vi "Main.vi"() -> ()   [LabVIEW 2021, in "Game of Life.lvlib"]
doc: "This template is for the Queued Message Handler design pattern.\n\nThe Event Handling Loop generates messages based on user interface actions.\n\nThe Message Handling Loop processes messages generated by the Event Handling Loop, or by other messages. The messages are string values, so new messages can be added easily to the Message Cases case structure in the Message Handling Loop. Each message cluster can also provide an optional value for Message Data, which is a variant that can be converted to whatever message-specific data is required."
uses:
  Game of Life.lvlib
  <vilib>/Plug-In SDKs/InstrumentStudio SDK/InstrumentStudioPluginSDK.lvlibp/Plugin Events Enum.ctl
  controls/Data.ctl
  controls/Configuration.ctl
  controls/Game of Life.ctl
  a2cd5499-92a9-455c-b0f9-1db12e3f6067.vi
  aef85ed4-6d5b-4a62-8cd4-232f16e6ae51.vi
  a2cd5499-92a9-455c-b0f9-1db12e3f6067.vi/6651a77e-856e-4bcd-af5a-c0c13b264cc1.vi
  aef85ed4-6d5b-4a62-8cd4-232f16e6ae51.vi/331b549c-fcf8-43d9-8a1e-5b3c0091a99c.vi
  <vilib>/JDP Science/JSONtext/JSON text to Variant.vi
  <vilib>/Utility/error.llb/Error Cluster From Error Code.vi
  <vilib>/JDP Science/JSONtext/Variant to JSON Text.vi
  <vilib>/JDP Science/JSONtext/LVClass Serializer/JSONtext LVClass Serializer.lvclass
  <vilib>/ErrorRing/Error Ring.xnode
  <vilib>/Plug-In SDKs/InstrumentStudio SDK/InstrumentStudioPluginSDK.lvlibp/Plugin Session.lvclass
  <vilib>/Plug-In SDKs/InstrumentStudio SDK/InstrumentStudioPluginSDK.lvlibp
panel:
  in  "Tab Control":enum32{"Game Panel", "Events"}(tab)
  in  "IS Project":bool
  in  "Start":bool
  out "game of life":T1(graph)
  out "generation":u32 caption="Generation"
  in  "update interval":u32=250 caption="Update interval (msec)" min=50
  in  "height":u32=100 caption="Board height" min=10
  in  "width":u32=100 caption="Board width" min=10
  out "Project Path":path
  out "Event Record":i32(listbox)
  in  "Session Id":u64
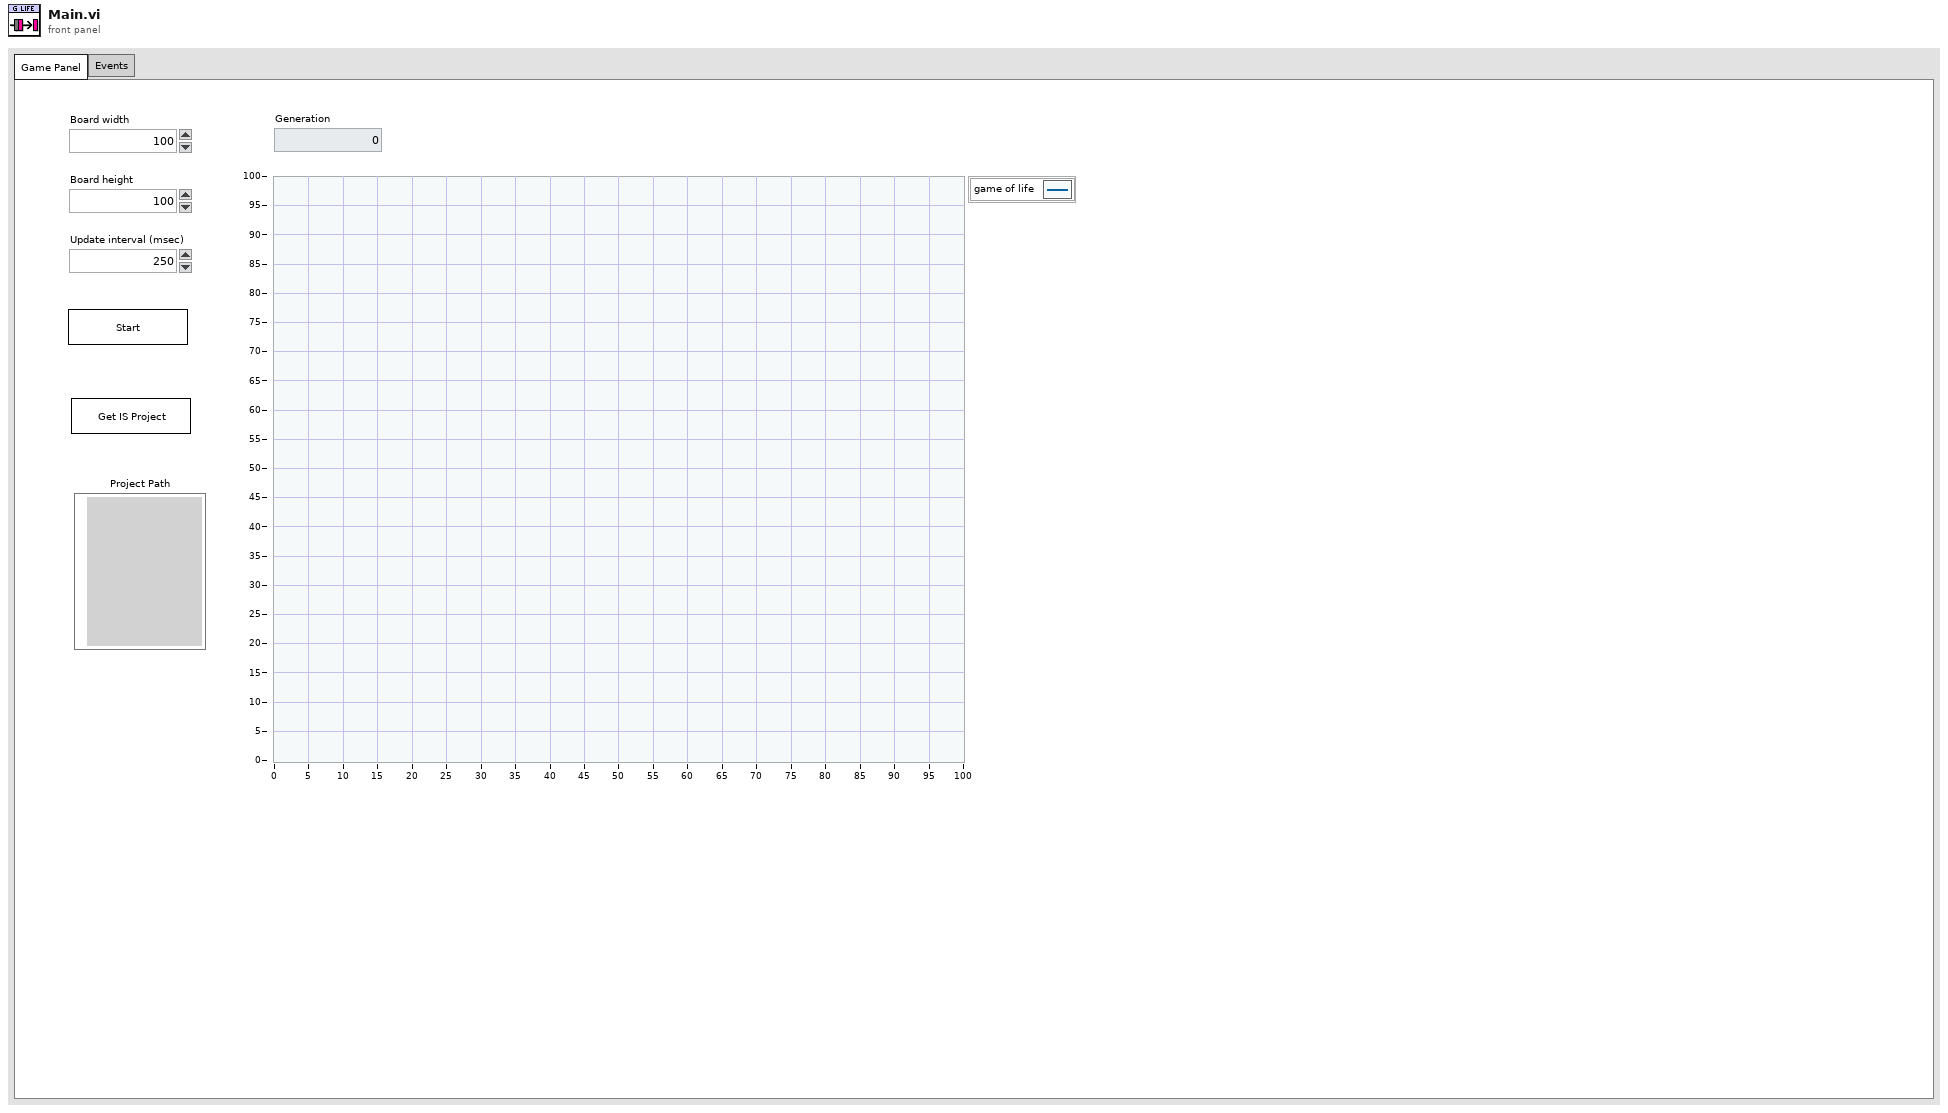
[diagram p1: front panel]
types:
  T1 = typedef "Game of Life.lvlib/Game of Life.ctl" = cluster{"x_data":dbl[], "y_data":dbl[]}
  T2 = typedef "Game of Life.lvlib/Data.ctl" = cluster{"Height":u32, "Width":u32, "Update Interval":u32, "Generation":u32, "Run?":bool, "Cells":bool[][], "Project Path":path}
  T3 = typedef "InstrumentStudioPluginSDK.lvlibp/Plugin Events Enum.ctl" = enum16{"Shutdown", "Project Saved", "Stop All Outputs"}
  T4 = typedef "InstrumentStudioPluginSDK.lvlibp/Event Registration Refnum.ctl" = refnum<event-registration>
  T5 = typedef "Game of Life.lvlib/All Message Queues.ctl" = cluster{"UI":refnum<queue>}
  T6 = cluster{"Event Refnum":T4, "Event Registration Refnum":refnum<event-registration>}
  T7 = typedef "Game of Life.lvlib/Configuration.ctl" = cluster{"Height":u32, "Width":u32, "Update Interval":u32, "Project Path":path}
  T8 = enum8{"Enabled", "Disabled", "Disabled and Grayed Out"}
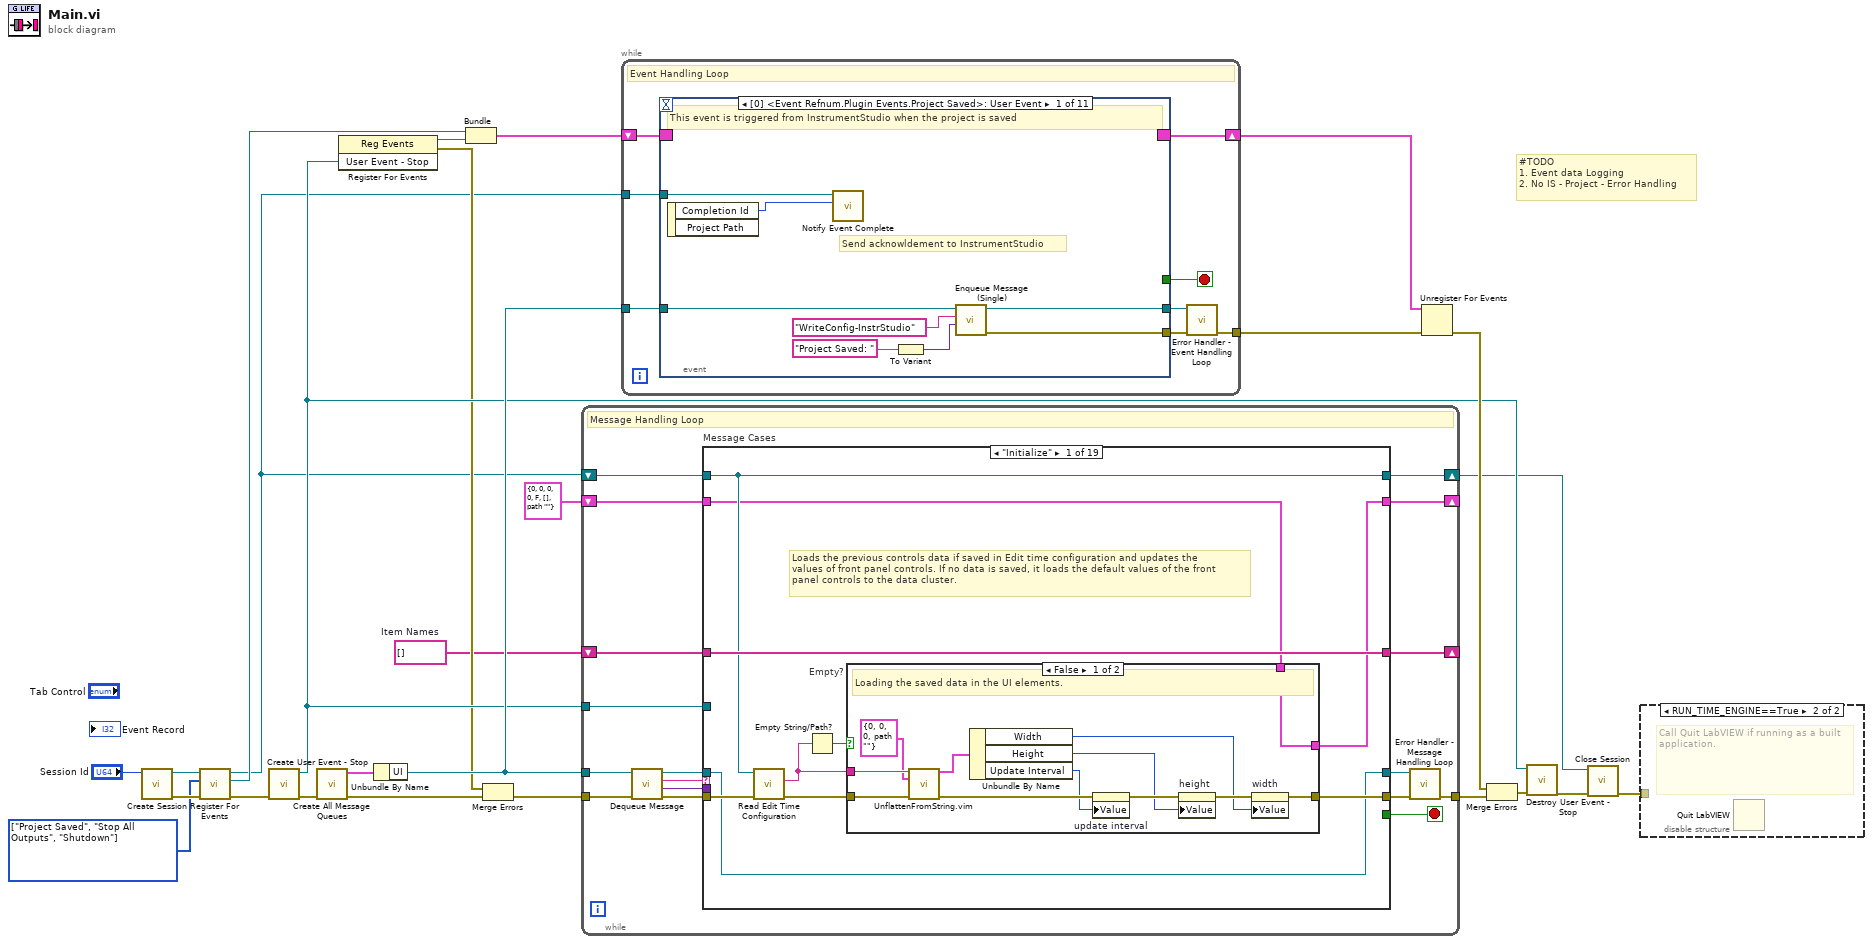
[diagram p0: block diagram]
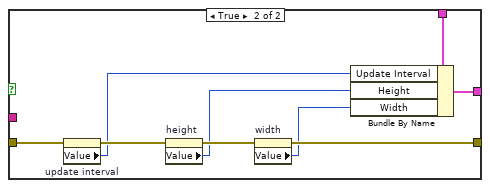
[diagram p3: hidden frame]
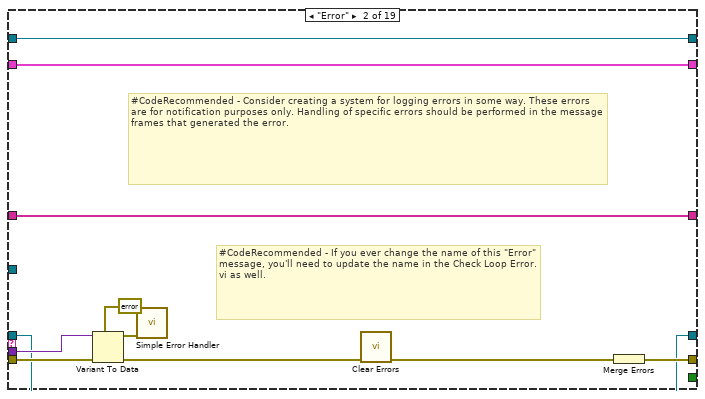
[diagram p4: hidden frame]
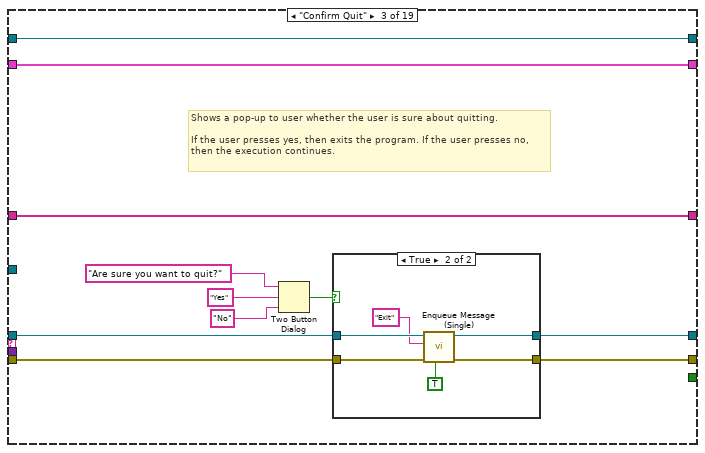
[diagram p5: hidden frame]
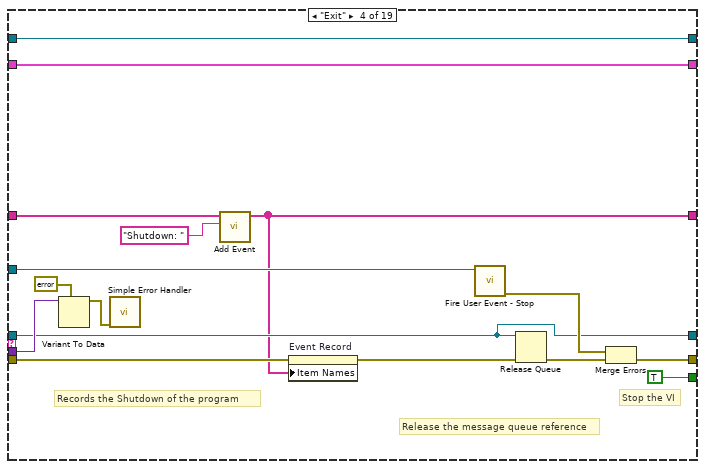
[diagram p7: hidden frame]
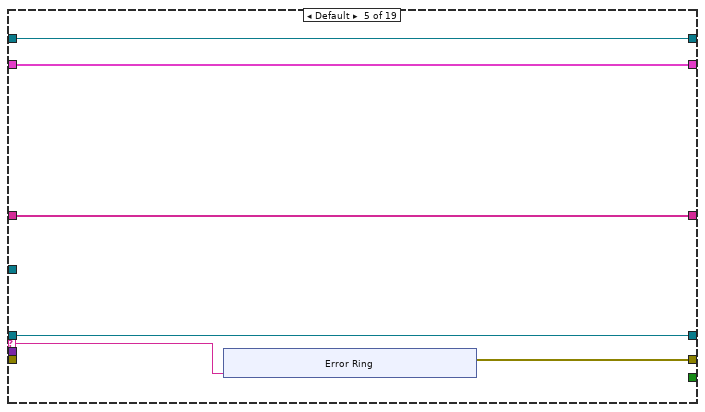
[diagram p8: hidden frame]
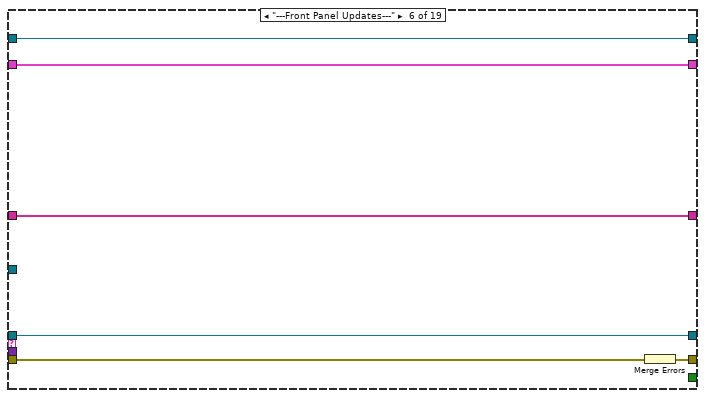
[diagram p9: hidden frame]
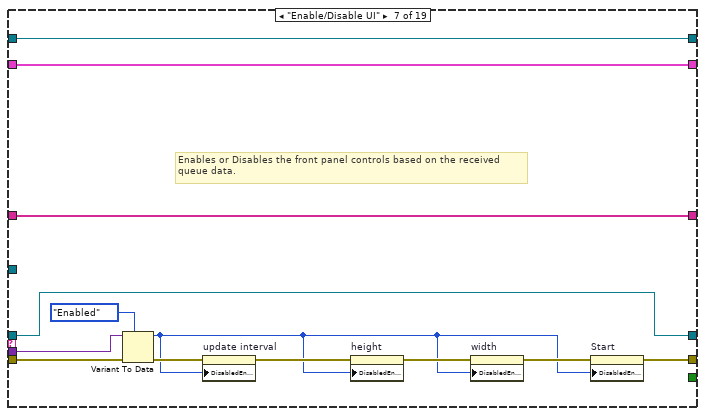
[diagram p10: hidden frame]
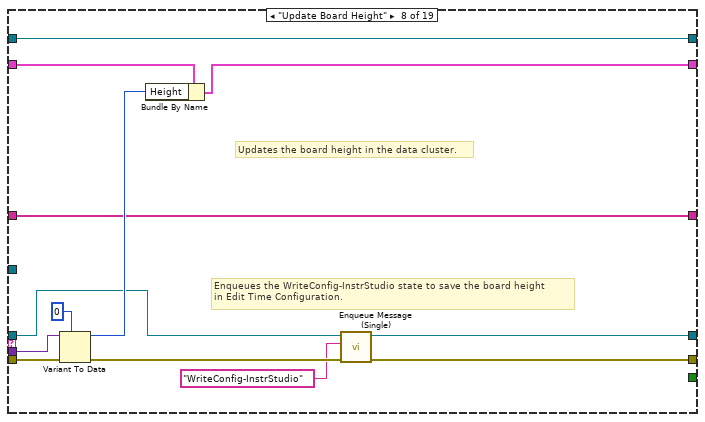
[diagram p11: hidden frame]
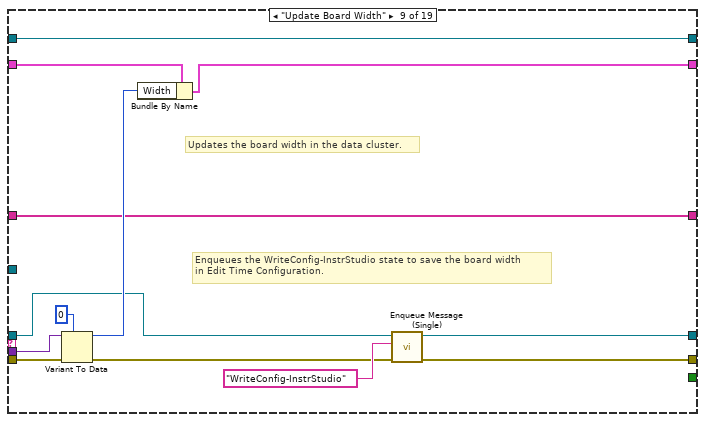
[diagram p12: hidden frame]
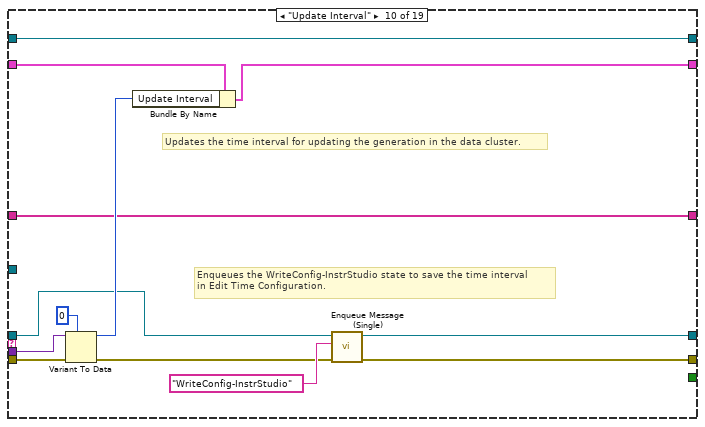
[diagram p13: hidden frame]
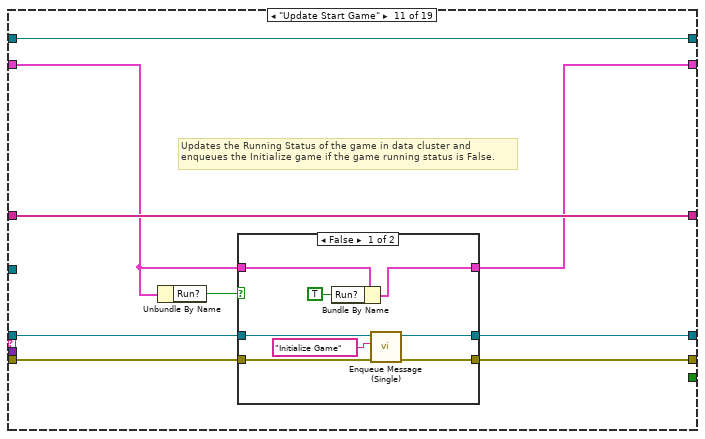
[diagram p14: hidden frame]
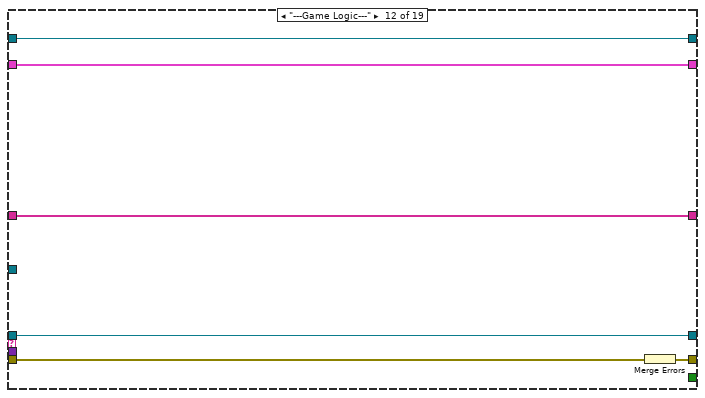
[diagram p16: hidden frame]
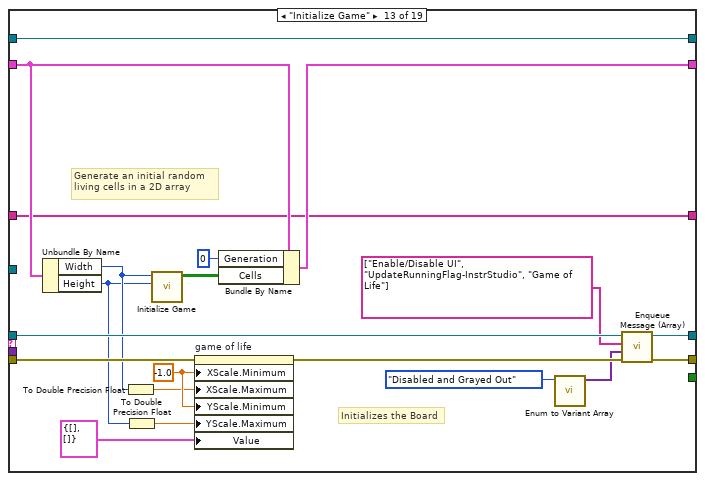
[diagram p17: hidden frame]
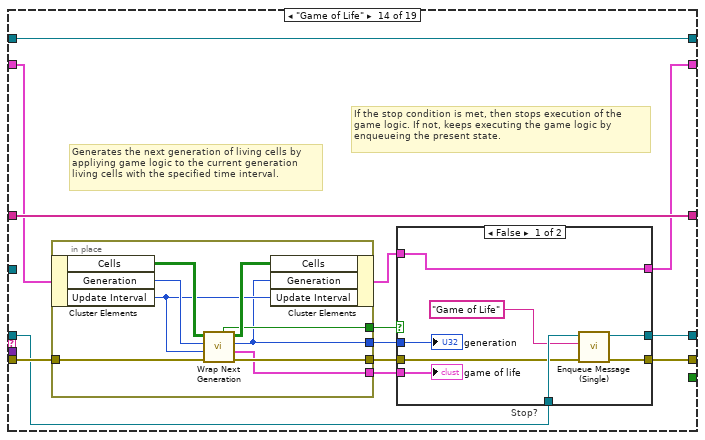
[diagram p18: hidden frame]
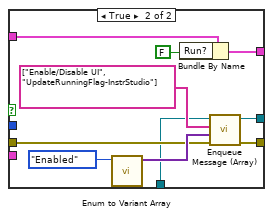
[diagram p19: hidden frame]
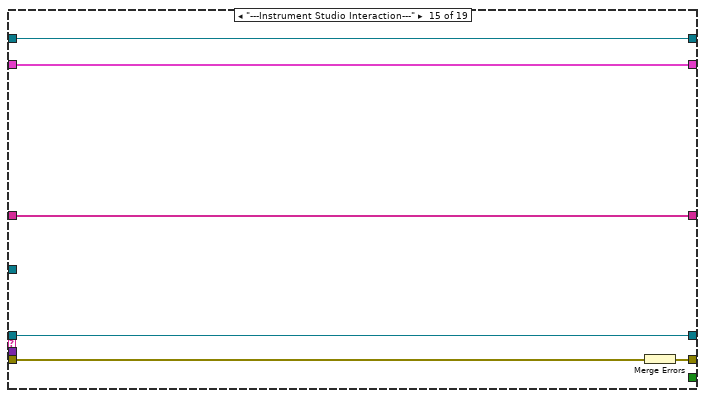
[diagram p20: hidden frame]
diagram:
  w1 = string[] []  # Item Names
  w10 = T3[] [enum."Project Saved", enum."Stop All Outputs", enum."Shutdown"] items=["Shutdown", "Project Saved", "Stop All Outputs"] ("Events To Register")
  # "#TODO\n1. Event data Logging\n2. No IS - Project - Error Handling"
  n1 = call <vilib>:"Create Session.vi"("Session Id"="Session Id") -> ("error out"=w13:errorcluster, "Session out"=w11:refnum<class "Plugin Session.lvclass">)  [unwired: 6 in, 3 out]
  n2 = call <vilib>:"Register For Events.vi"("error in (no error)"=w13, "Events To Register"=w10, "Session in"=w11) -> ("error out"=w12:errorcluster, "Event Refnum"=w7:T4, "Session out"=w3:refnum<class "Plugin Session.lvclass">)  [unwired: 6 in]
  n3 = call "Create User Event - Stop.vi"("error in (no error)"=w12) -> ("error out"=w22:errorcluster, "User Event - Stop"=w17:refnum<user-event>)  [unwired: 9 in]
  n4 = call "Create All Message Queues.vi"("error in (no error)"=w22) -> ("error out"=w26:errorcluster, "Message Queues out"=w25:T5)  [unwired: 9 in]
  n5 = register-events(w17) -> (reference out=w9:refnum<event-registration>, error out=w15:errorcluster)  [unwired: 2 in]
  n6 = Unbundle By Name(w25) -> ("UI"=w23:refnum<queue>)
  n7 = Bundle("Event Refnum"=w7, "Event Registration Refnum"=w9) -> (w8:T6)  [unwired: 1 in]
  n8 = Merge Errors(w15, w26) -> (w16:errorcluster)
  n9 = while {
    tunnel: w23 -> [w37]
    tunnel: w17 -> [w42]
    tunnel: w16 -> [w41]
    tunnel: [w35] -> w24
    shift-right: [w32] -> w6
    shift-left: w3 -> [w33]
    shift-right: [w31] -> _
    shift-left: T2 {"Height"=0, "Width"=0, "Update Interval"=0, "Generation"=0, "Run?"=FALSE, "Cells"=[], "Project Path"=path ""} ("Configuration") -> [w30]
    shift-right: [w28] -> _
    shift-left: w1 -> [w29]
    stop <- w43 stop-if-true
    # "Message Handling Loop"
    n10 = call "Dequeue Message.vi"("error in (no error)"=w41, "Message Queue"=w37) -> ("error out"=w40:errorcluster, "Message Data"=w38:variant, "Message"=w39:string, "dup Message Queue"=w36:refnum<queue>)  [unwired: 6 in]
    n11 = case "Message Cases" shown="\"Initialize\"" w39 {
      selector: w39 -> [_ _ _ _ w125 _ _ _ _ _ _ _ _ _ _ _ _ _ _]
      tunnel: w36 -> [w46 w75 w94 w110 w121 w134 w141 w154 w167 w179 w193 w212 w231 w244 w278 w294 w303 w310 w323]
      tunnel: w40 -> [w49 w85 w96 w108 _ w139 w145 w164 w177 w190 w199 w217 w229 w249 w283 w296 w305 w316 w322]
      tunnel: [w53 w80 w95 w118 w126 w138 w147 w156 w166 w181 w194 w216 w232 w245 w282 w292 w306 w314 w335] -> w34
      tunnel: [_ _ _ TRUE _ _ _ _ _ _ _ _ _ _ _ _ _ _ _] -> w43
      tunnel: w38 -> [_ w84 _ w113 _ _ w144 w163 w176 w189 _ _ _ _ _ _ _ _ w320]
      tunnel: w42 -> [_ _ _ w117 _ _ _ _ _ _ _ _ _ _ _ _ _ _ _]
      tunnel: w33 -> [w47 w79 w93 w112 w124 w137 w152 w165 w178 w191 w200 w215 w237 w250 w281 w300 w308 w317 w337]
      tunnel: [w47 w79 w93 w112 w124 w137 w152 w165 w178 w191 w200 w215 w237 w250 w281 w300 w307 w315 w336] -> w32
      tunnel: [w45 w78 w92 w111 w123 w136 w151 w160 w174 w187 w195 w214 w236 w238 w280 w298 w302 w312 w329] -> w31
      tunnel: w30 -> [w44 w78 w92 w111 w123 w136 w151 w159 w173 w186 w196 w214 w235 w242 w280 w297 w302 w311 w329]
      tunnel: w29 -> [w48 w76 w91 w107 w122 w135 w140 w158 w171 w184 w198 w213 w234 w248 w279 w288 w304 w313 w321]
      tunnel: [w48 w76 w91 w106 w122 w135 w140 w158 w171 w184 w198 w213 w234 w248 w279 w289 w304 w313 w331] -> w28
      tunnel: [w46 w75 w90 w110 w121 w134 w141 w155 w168 w180 w192 w212 w230 w241 w278 w290 w303 w310 w323] -> w27
      frame "Initialize" {
        # "Loads the previous controls data if saved in Edit time configuration and updates the\nvalues of front panel controls. If no data is saved, it loads the default values of the front\npanel controls to the data cluster."
        # "Initialize - All initialization work should take place in this message, since other loops can potentially enqueue messages that execute immediately after this one."
        n12 = call <vilib>:"Read Edit Time Configuration.vi"("error in (no error)"=w49, "Session in"=w47) -> ("error out"=w50:errorcluster, "Edit Time Configuration"=w51:string)  [unwired: 7 in, 1 out]
        n13 = Empty String/Path?(string/path=w51) -> (empty?=w52:bool)
        n14 = case "Empty?" shown="False" w52 {
          tunnel: [w57 w71] -> w53
          tunnel: w50 -> [w64 w70]
          tunnel: w51 -> [w65 _]
          tunnel: w44 -> [w54 w74]
          tunnel: [w54 w68] -> w45
          frame False {
            # "Loading the saved data in the UI elements."
            n15 = call "UnflattenFromString.vim"("Flattened Data"=w65, "Data Type"=T7 {"Height"=0, "Width"=0, "Update Interval"=0, "Project Path"=path ""} ("Configuration"), "error in"=w64) -> ("Data Out"=w63:T7, "error out"=w62:errorcluster)  [unwired: 11 in]
            n16 = Unbundle By Name(w63) -> ("Width"=w56:u32, "Height"=w59:u32, "Update Interval"=w61:u32)
            n17 = property on="update interval" class="DigNum (strict)"(error in=w62, "Value"=w61) -> (error out=w60:errorcluster)  [unwired: 1 in, 1 out]
            n18 = property on="height" class="DigNum (strict)"(error in=w60, "Value"=w59) -> (error out=w58:errorcluster)  [unwired: 1 in, 1 out]
            n19 = property on="width" class="DigNum (strict)"(error in=w58, "Value"=w56) -> (error out=w57:errorcluster)  [unwired: 1 in, 1 out]
          }
          frame True {
            n20 = property on="update interval" class="DigNum (strict)"(error in=w70) -> (error out=w73:errorcluster, "Value"=w69:u32)  [unwired: 1 in, 1 out]
            n21 = property on="height" class="DigNum (strict)"(error in=w73) -> (error out=w72:errorcluster, "Value"=w67:u32)  [unwired: 1 in, 1 out]
            n22 = property on="width" class="DigNum (strict)"(error in=w72) -> (error out=w71:errorcluster, "Value"=w66:u32)  [unwired: 1 in, 1 out]
            n23 = Bundle By Name(cluster=w74, "Update Interval"=w69, "Height"=w67, "Width"=w66) -> (w68:T2)
          }
        }
      }
      frame "Error" {
        # "#CodeRecommended - If you ever change the name of this \"Error\" message, you'll need to update the name in the Check Loop Error.vi as well."
        # "#CodeRecommended - Consider creating a system for logging errors in some way. These errors are for notification purposes only. Handling of specific errors should be performed in the message frames that generated the error."
        # "Error - Display an error dialog. This message is sent by the \"Error Handler\" VIs at the end of other loops in this application."
        n24 = Variant To Data(error in=w85, type=errorcluster {"status"=FALSE, "code"=0, "source"=""} ("error constant"), Variant=w84) -> (data=w82:errorcluster, error out=w81:errorcluster)
        n25 = call <vilib>:"Simple Error Handler.vi"("error in (no error)"=w82) -> ()  [unwired: 4 in, 5 out]
        n26 = call <vilib>:"Clear Errors.vi"("error in (no error)"=w81) -> ("error out"=w77:errorcluster)  [unwired: 5 in, 1 out]
        n27 = Merge Errors(w77) -> (w80:errorcluster)
      }
      frame "Confirm Quit" {
        # "Shows a pop-up to user whether the user is sure about quitting. \n\nIf the user presses yes, then exits the program. If the user presses no,\nthen the execution continues."
        # "Confirm Quit - Message that can confirm whether or not the user wants to exit the application."
        n28 = Two Button Dialog(message="Are sure you want to quit?", 1:"No" ("F button name (\"Cancel\")"), 2:"Yes" ("T button name (\"OK\")")) -> (T button?=w86:bool)
        n29 = case shown="True" w86 {
          tunnel: w96 -> [w97 w104]
          tunnel: [w97 w103] -> w95
          tunnel: w94 -> [w98 w102]
          tunnel: [w98 w99] -> w90
          frame False {
          }
          frame True {
            n30 = call "Enqueue Message (Single).vi"("Priority Message? (F)"=TRUE, "error in (no error)"=w104, "Message"="Exit", "Message Queue"=w102) -> ("error out"=w103:errorcluster, "dup Message Queue"=w99:refnum<queue>)  [unwired: 6 in]
          }
        }
      }
      frame "Exit" {
        # "Records the Shutdown of the program"
        # "Stop the VI"
        # "Release the message queue reference"
        # "Exit - Exit the application."
        n31 = Variant To Data(type=errorcluster {"status"=FALSE, "code"=0, "source"=""} ("error constant"), Variant=w113) -> (data=w114:errorcluster)  [unwired: 1 in, 1 out]
        n32 = call <vilib>:"Simple Error Handler.vi"("error in (no error)"=w114) -> ()  [unwired: 4 in, 5 out]
        n33 = call "Add Event.vi"("Event Tag"="Shutdown: ", "Item Names in"=w107) -> ("Item Names out"=w106:string[])  [unwired: 9 in]
        n34 = property on="Event Record" class="LstBox (strict)"(error in=w108, "Item Names"=w106) -> (error out=w109:errorcluster)  [unwired: 1 in, 1 out]
        n35 = call "Fire User Event - Stop.vi"("User Event - Stop"=w117) -> ("error out"=w116:errorcluster)  [unwired: 10 in]
        n36 = Release Queue(queue=w110, error in (no error)=w109) -> (error out=w119:errorcluster)  [unwired: 1 in, 2 out]
        n37 = Merge Errors(w116, w119) -> (w118:errorcluster)
      }
      frame Default {
        # "'Default' case only runs if there is a message that isn't defined in any of the other cases.  Output a programming error."
        n38 = xnode "Error Ring"("parameter 0"=w125) -> ("error out"=w126:errorcluster)
      }
      frame "---Front Panel Updates---" {
        # "Duplicate this frame when creating new messages.  Change this comment in the duplicated frame to describe this message."
        n39 = Merge Errors(w139) -> (w138:errorcluster)
      }
      frame "Enable/Disable UI" {
        # "Enables or Disables the front panel controls based on the received \nqueue data."
        n40 = Variant To Data(error in=w145, type=T8."Enabled" ("Disabled"), Variant=w144) -> (data=w142:T8, error out=w146:errorcluster)
        n41 = property on="update interval" class="DigNum (strict)"(error in=w146, "DisabledEnum"=w142) -> (error out=w150:errorcluster)  [unwired: 1 in, 1 out]
        n42 = property on="height" class="DigNum (strict)"(error in=w150, "DisabledEnum"=w142) -> (error out=w149:errorcluster)  [unwired: 1 in, 1 out]
        n43 = property on="width" class="DigNum (strict)"(error in=w149, "DisabledEnum"=w142) -> (error out=w148:errorcluster)  [unwired: 1 in, 1 out]
        n44 = property on="Start" class="Bool"(error in=w148, "DisabledEnum"=w142) -> (error out=w147:errorcluster)  [unwired: 1 in, 1 out]
      }
      frame "Update Board Height" {
        # "Enqueues the WriteConfig-InstrStudio state to save the board height\nin Edit Time Configuration."
        # "Updates the board height in the data cluster."
        n45 = Variant To Data(error in=w164, type=u32 0 ("wid"), Variant=w163) -> (data=w161:u32, error out=w157:errorcluster)
        n46 = Bundle By Name(cluster=w159, "Height"=w161) -> (w160:T2)
        n47 = call "Enqueue Message (Single).vi"("error in (no error)"=w157, "Message"="WriteConfig-InstrStudio", "Message Queue"=w154) -> ("error out"=w156:errorcluster, "dup Message Queue"=w155:refnum<queue>)  [unwired: 7 in]
      }
      frame "Update Board Width" {
        # "Enqueues the WriteConfig-InstrStudio state to save the board width\nin Edit Time Configuration."
        # "Updates the board width in the data cluster."
        n48 = Variant To Data(error in=w177, type=u32 0 ("wid"), Variant=w176) -> (data=w172:u32, error out=w169:errorcluster)
        n49 = Bundle By Name(cluster=w173, "Width"=w172) -> (w174:T2)
        n50 = call "Enqueue Message (Single).vi"("error in (no error)"=w169, "Message"="WriteConfig-InstrStudio", "Message Queue"=w167) -> ("error out"=w166:errorcluster, "dup Message Queue"=w168:refnum<queue>)  [unwired: 7 in]
      }
      frame "Update Interval" {
        # "Enqueues the WriteConfig-InstrStudio state to save the time interval\nin Edit Time Configuration."
        # "Updates the time interval for updating the generation in the data cluster."
        n51 = Variant To Data(error in=w190, type=u32 0 ("wid"), Variant=w189) -> (data=w185:u32, error out=w182:errorcluster)
        n52 = Bundle By Name(cluster=w186, "Update Interval"=w185) -> (w187:T2)
        n53 = call "Enqueue Message (Single).vi"("error in (no error)"=w182, "Message"="WriteConfig-InstrStudio", "Message Queue"=w179) -> ("error out"=w181:errorcluster, "dup Message Queue"=w180:refnum<queue>)  [unwired: 7 in]
      }
      frame "Update Start Game" {
        # "Updates the Running Status of the game in data cluster and\nenqueues the Initialize game if the game running status is False."
        n54 = Unbundle By Name(w196) -> ("Run?"=w197:bool)
        n55 = case shown="False" w197 {
          tunnel: w199 -> [w203 w210]
          tunnel: w196 -> [w208 w211]
          tunnel: [w207 w211] -> w195
          tunnel: [w204 w210] -> w194
          tunnel: w193 -> [w205 w209]
          tunnel: [w202 w209] -> w192
          frame False {
            n56 = Bundle By Name(cluster=w208, "Run?"=TRUE) -> (w207:T2)
            n57 = call "Enqueue Message (Single).vi"("error in (no error)"=w203, "Message"="Initialize Game", "Message Queue"=w205) -> ("error out"=w204:errorcluster, "dup Message Queue"=w202:refnum<queue>)  [unwired: 7 in]
          }
          frame True {
          }
        }
      }
      frame "---Game Logic---" {
        # "Duplicate this frame when creating new messages.  Change this comment in the duplicated frame to describe this message."
        n58 = Merge Errors(w217) -> (w216:errorcluster)
      }
      frame "Initialize Game" {
        w228 = -1.0 ("X Scale.Range:Minimum")
        # "Generate an initial random \nliving cells in a 2D array"
        # "Initializes the Board"
        n59 = Unbundle By Name(w235) -> ("Width"=w226:u32, "Height"=w224:u32)
        n60 = To Double Precision Float(number=w226) -> (double precision float=w227:dbl)
        n61 = To Double Precision Float(number=w224) -> (double precision float=w225:dbl)
        n62 = call "Initialize Game.vi"("Height"=w224, "Width"=w226) -> ("Array"=w233:bool[][])  [unwired: 9 in]
        n63 = property on="game of life" class="XYGraph (strict)"(error in=w229, "XScale.Minimum"=w228, "XScale.Maximum"=w227, "YScale.Minimum"=w228, "YScale.Maximum"=w225, "Value"=T1 {"x_data"=[], "y_data"=[]} ("game of life")) -> (error out=w223:errorcluster)  [unwired: 1 in, 1 out]
        n64 = Bundle By Name(cluster=w235, "Generation"=u32 0, "Cells"=w233) -> (w236:T2)
        n65 = call "Enum to Variant Array.vi"("Disabled"=T8."Disabled and Grayed Out") -> ("Message Data Array"=w218:variant[])  [unwired: 10 in]
        n66 = call "Enqueue Message (Array).vi"("error in (no error)"=w223, "Message Data Array"=w218, "Message Array"=string[] ["Enable/Disable UI", "UpdateRunningFlag-InstrStudio", "Game of Life"], "Message Queue"=w231) -> ("error out"=w232:errorcluster, "dup Message Queue"=w230:refnum<queue>)  [unwired: 6 in]
      }
      frame "Game of Life" {
        # "If the stop condition is met, then stops execution of the \ngame logic. If not, keeps executing the game logic by \nenqueueing the present state."
        # "Generates the next generation of living cells by\nappliying game logic to the current generation \nliving cells with the specified time interval."
        n67 = in-place {
          in-place-border: w249 -> [w259]
          in-place-border: [w255] -> w246
          in-place-border: [w254] -> w247
          in-place-border: [w253] -> w243
          in-place-border: [w251] -> w240
          n68 = in-place-cluster #1(w242) -> ("Cells"=w258:bool[][], "Generation"=w257:u32, "Update Interval"=w252:u32)
          n69 = call "Wrap Next Generation.vi"("error in"=w259, "Update Interval"=w252, "generation in"=w257, "cells in"=w258) -> ("error out"=w255:errorcluster, "game of life"=w253:T1, "generation out"=w251:u32, "cells out"=w256:bool[][], "Stop?"=w254:bool)  [unwired: 3 in]
          n70 = in-place-cluster #1("Cells"=w256, "Generation"=w251, "Update Interval"=w252) -> (w239:T2)
        }
        n71 = case "Stop?" shown="False" w247 {
          tunnel: w246 -> [w264 w273]
          tunnel: [w267 w274] -> w245
          tunnel: w244 -> [w266 w272]
          tunnel: w243 -> [w261 _]
          tunnel: [w263 w271] -> w241
          tunnel: w240 -> [w262 _]
          tunnel: w239 -> [w260 w269]
          tunnel: [w260 w270] -> w238
          frame False {
            n72 = call "Enqueue Message (Single).vi"("error in (no error)"=w264, "Message"="Game of Life", "Message Queue"=w266) -> ("error out"=w267:errorcluster, "dup Message Queue"=w263:refnum<queue>)  [unwired: 7 in]
            "generation" <- w262
            "game of life" <- w261
          }
          frame True {
            n73 = call "Enum to Variant Array.vi"("Disabled"=T8."Enabled") -> ("Message Data Array"=w277:variant[])  [unwired: 10 in]
            n74 = Bundle By Name(cluster=w269, "Run?"=FALSE) -> (w270:T2)
            n75 = call "Enqueue Message (Array).vi"("error in (no error)"=w273, "Message Data Array"=w277, "Message Array"=string[] ["Enable/Disable UI", "UpdateRunningFlag-InstrStudio"], "Message Queue"=w272) -> ("error out"=w274:errorcluster, "dup Message Queue"=w271:refnum<queue>)  [unwired: 6 in]
          }
        }
      }
      frame "---Instrument Studio Interaction---" {
        # "Duplicate this frame when creating new messages.  Change this comment in the duplicated frame to describe this message."
        n76 = Merge Errors(w283) -> (w282:errorcluster)
      }
      frame "StopAllOutputs" {
        # "Flush the Queue to stop game logic execution"
        # "Updates the Running Status of the game in data cluster"
        # "Updates the Event Record indicator with current event."
        n77 = call "Add Event.vi"("Event Tag"="Stop All Outputs: ", "Item Names in"=w288) -> ("Item Names out"=w289:string[])  [unwired: 9 in]
        n78 = property on="Event Record" class="LstBox (strict)"(error in=w296, "Item Names"=w289) -> (error out=w295:errorcluster)  [unwired: 1 in, 1 out]
        n79 = Bundle By Name(cluster=w297, "Run?"=FALSE) -> (w298:T2)
        n80 = Flush Queue(queue=w294, error in (no error)=w295) -> (queue out=w291:refnum<queue>, error out=w293:errorcluster)  [unwired: 1 out]
        n81 = call "Enum to Variant Array.vi"("Disabled"=T8."Enabled") -> ("Message Data Array"=w285:variant[])  [unwired: 10 in]
        n82 = call "Enqueue Message (Array).vi"("error in (no error)"=w293, "Message Data Array"=w285, "Message Array"=string[] ["Enable/Disable UI", "UpdateRunningFlag-InstrStudio"], "Message Queue"=w291) -> ("error out"=w292:errorcluster, "dup Message Queue"=w290:refnum<queue>)  [unwired: 6 in]
      }
      frame "UpdateRunningFlag-InstrStudio" {
        # "Updates the running flag in \nInstrumentStudio"
        n83 = Unbundle By Name(w302) -> ("Run?"=w301:bool)
        n84 = call <vilib>:"Update Running State.vi"("error in (no error)"=w305, "Is Running"=w301, "Plugin Session in"=w308) -> ("error out"=w306:errorcluster, "Plugin Session out"=w307:refnum<class "Plugin Session.lvclass">)  [unwired: 7 in]
      }
      frame "ReadISProjectPath" {
        # "#TODO\nEvent Logging"
        # "Reads the InstrumentStudio project path"
        n85 = call <vilib>:"Read Project Path.vi"("error in (no error)"=w316, "Session in"=w317) -> ("error out"=w314:errorcluster, "Project Path"=w309:path, "Session out"=w315:refnum<class "Plugin Session.lvclass">)  [unwired: 7 in]
        "Project Path" <- w309
        n86 = Bundle By Name(cluster=w311, "Project Path"=w309) -> (w312:T2)
      }
      frame "WriteConfig-InstrStudio" {
        # "Saving the control inputs\nin the instrumentStudio object"
        n87 = Equal?(x=w320, y=variant) -> (x = y?=w318:bool)
        n88 = case "Empty Variant?" shown="False" w318 {
          tunnel: [w345 w346] -> w332
          tunnel: [w344 w347] -> w331
          tunnel: w322 -> [w340 w346]
          tunnel: w320 -> [w339 _]
          tunnel: w321 -> [w343 w347]
          frame False {
            # "Records the project save event in event record indicator."
            n89 = Variant To Data(error in=w340, type="", Variant=w339) -> (data=w338:string, error out=w341:errorcluster)
            n90 = call "Add Event.vi"("Event Tag"=w338, "Item Names in"=w343) -> ("Item Names out"=w344:string[])  [unwired: 9 in]
            n91 = property on="Event Record" class="LstBox (strict)"(error in=w341, "Item Names"=w344) -> (error out=w345:errorcluster)  [unwired: 1 in, 1 out]
          }
          frame True {
          }
        }
        n92 = Unbundle By Name(w329) -> ("Height"=w328:u32, "Width"=w327:u32, "Update Interval"=w326:u32, "Project Path"=w325:path)
        n93 = Bundle By Name(cluster=T7 {"Height"=0, "Width"=0, "Update Interval"=0, "Project Path"=path ""} ("Configuration"), "Height"=w328, "Width"=w327, "Update Interval"=w326, "Project Path"=w325) -> (w324:T7)
        n94 = call "FlattenToString.vim"("Anything"=w324, "error in"=w332) -> ("Flattened Data"=w334:string, "error out"=w333:errorcluster)  [unwired: 12 in]
        n95 = call <vilib>:"Write Edit Time Configuration.vi"("error in (no error)"=w333, "Edit Time Configuration"=w334, "Session in"=w337) -> ("error out"=w335:errorcluster, "Session out"=w336:refnum<class "Plugin Session.lvclass">)  [unwired: 7 in]
      }
    }
    n96 = call "Error Handler - Message Handling Loop.vi"("error in (no error)"=w34, "Message Queue"=w27) -> ("dup error in"=w35:errorcluster)  [unwired: 8 in, 1 out]
  }
  n97 = while {
    tunnel: w23 -> [w355]
    shift-right: [w353] -> w19
    shift-left: w8 -> [w354]
    tunnel: [w349] -> w18
    tunnel: w3 -> [w348]
    stop <- w351 stop-if-true
    # "Event Handling Loop"
    n98 = event shown="[0] <Event Refnum.Plugin Events.Project Saved>: User Event" {
      selector: w354 -> [_ _ _ _ _ _ _ _ _ _ _]
      dyn-events: [_ _ _ _ _ _ _ _ _ _ _] -> w353
      timeout: _ -> [_ _ _ _ _ _ _ _ _ _ _]
      tunnel: [_ _ _ _ _ _ _ _ _ TRUE ("Discard?") _] -> w351
      tunnel: w355 -> [w360 w368 w371 w379 w385 w391 w395 w402 w404 w406 w409]
      tunnel: [w358 w365 w372 w378 w384 w390 w394 w401 _ _ w407] -> w352
      tunnel: [w359 w366 w373 w380 w386 w392 w396 w400 w404 w406 w410] -> w350
      tunnel: w348 -> [w363 w370 _ _ _ _ _ _ _ _ _]
      event User Event {
        # "Send acknowldement to InstrumentStudio"
        # "This event is triggered from InstrumentStudio when the project is saved"
        n99 = event-data() -> ("Completion Id"=w362:i64)  [unwired: 1 in, 1 out]
        n100 = call <vilib>:"Notify Event Complete.vi"("Completion Id"=w362, "Session in"=w363) -> ()  [unwired: 8 in, 2 out]
        n101 = To Variant(anything="Project Saved: " ("string")) -> (Variant=w357:variant)
        n102 = call "Enqueue Message (Single).vi"("Message Data"=w357, "Message"="WriteConfig-InstrStudio", "Message Queue"=w360) -> ("error out"=w358:errorcluster, "dup Message Queue"=w359:refnum<queue>)  [unwired: 7 in]
      }
      event User Event {
        # "Send acknowldement to InstrumentStudio"
        # "This event is triggered from InstrumentStudio when the project Stop All Outputs button is pressed"
        n103 = event-data() -> ("Completion Id"=w369:i64)  [unwired: 1 in]
        n104 = call <vilib>:"Notify Event Complete.vi"("Completion Id"=w369, "Session in"=w370) -> ()  [unwired: 8 in, 2 out]
        n105 = call "Enqueue Message (Single).vi"("Priority Message? (F)"=TRUE, "Message"="StopAllOutputs", "Message Queue"=w368) -> ("error out"=w365:errorcluster, "dup Message Queue"=w366:refnum<queue>)  [unwired: 7 in]
      }
      event User Event {
        # "This event doesn't need acknowledgement from plugin"
        # "This event is triggered when softpanel/instrumentstudio is closed"
        n106 = event-data() -> ()  [unwired: 1 in, 1 out]
        n107 = call "Enqueue Message (Single).vi"("Priority Message? (F)"=TRUE, "Message"="Exit", "Message Queue"=w371) -> ("error out"=w372:errorcluster, "dup Message Queue"=w373:refnum<queue>)  [unwired: 7 in]
      }
      event "height": Value Change {
        # "Captures value change in height and sends data to Message Handling Loop"
        n108 = event-data() -> ("NewVal"=w377:u32)  [unwired: 1 in]
        n109 = To Variant(anything=w377) -> (Variant=w376:variant)
        n110 = call "Enqueue Message (Single).vi"("Message Data"=w376, "Message"="Update Board Height", "Message Queue"=w379) -> ("error out"=w378:errorcluster, "dup Message Queue"=w380:refnum<queue>)  [unwired: 7 in]
      }
      event "width": Value Change {
        # "Captures value change in width and sends data to Message Handling Loop"
        n111 = event-data() -> ("NewVal"=w383:u32)  [unwired: 1 in]
        n112 = To Variant(anything=w383) -> (Variant=w382:variant)
        n113 = call "Enqueue Message (Single).vi"("Message Data"=w382, "Message"="Update Board Width", "Message Queue"=w385) -> ("error out"=w384:errorcluster, "dup Message Queue"=w386:refnum<queue>)  [unwired: 7 in]
      }
      event "update interval": Value Change {
        # "Captures value change in update interval and sends data to Message Handling Loop"
        n114 = event-data() -> ("NewVal"=w389:u32)  [unwired: 1 in]
        n115 = To Variant(anything=w389) -> (Variant=w388:variant)
        n116 = call "Enqueue Message (Single).vi"("Message Data"=w388, "Message"="Update Interval", "Message Queue"=w391) -> ("error out"=w390:errorcluster, "dup Message Queue"=w392:refnum<queue>)  [unwired: 7 in]
      }
      event "Start": Value Change {
        # "Captures value change in height and enqueues a state for Message Handling Loop"
        n117 = event-data() -> ()  [unwired: 1 in, 1 out]
        n118 = call "Enqueue Message (Single).vi"("Message"="Update Start Game", "Message Queue"=w395) -> ("error out"=w394:errorcluster, "dup Message Queue"=w396:refnum<queue>)  [unwired: 8 in]
      }
      event Panel Close? {
        # "Send the 'Confirm Quit' message if the user closes the panel of the VI. Discard the event so the 'Confirm Quit' message has a chance to run."
        n119 = event-data() -> ()  [unwired: 1 in, 1 out]
        n120 = call-poly "Enqueue Message.vi"("Priority Message? (F)"=TRUE, "Message"="Confirm Quit", "Message Queue"=w402) -> ("error out"=w401:errorcluster, "dup Message Queue"=w400:refnum<queue>)  [unwired: 7 in]
        n121 = event-data("Discard?"=TRUE) -> ()  [unwired: 1 in, 1 out]
      }
      event Application Instance Close {
        # "#CodeRecommended - When a project closes, all VIs within that project are aborted and leave memory. However, any code placed in this event frame is guaranteed to run to completion, so add any cleanup code that absolutely must happen here."
        n122 = event-data() -> ()  [unwired: 1 in, 1 out]
      }
      event User Event {
        # "The Message Handling Loop processed an \"Exit\" message, which fired this event to stop the Event Handling Loop."
        n123 = event-data() -> ()  [unwired: 1 in, 1 out]
      }
      event "IS Project": Value Change {
        # "#TODO\nEvent Logging"
        n124 = event-data() -> ()  [unwired: 1 in, 1 out]
        n125 = call "Enqueue Message (Single).vi"("Message"="ReadISProjectPath", "Message Queue"=w409) -> ("error out"=w407:errorcluster, "dup Message Queue"=w410:refnum<queue>)  [unwired: 8 in]
      }
    }
    n126 = call "Error Handler - Event Handling Loop.vi"("error in (no error)"=w352, "Message Queue"=w350) -> ("dup error in"=w349:errorcluster)  [unwired: 8 in, 1 out]
  }
  n127 = Unregister For Events(event registration refnum=w19, error in=w18) -> (error out=w20:errorcluster)
  n128 = Merge Errors(w20, w24) -> (w21:errorcluster)
  n129 = call "Destroy User Event - Stop.vi"("error in (no error)"=w21, "User Event - Stop"=w17) -> ("error out"=w5:errorcluster)  [unwired: 9 in]
  n130 = call <vilib>:"Close Session.vi"("error in (no error)"=w5, "Session in"=w6) -> ("error out"=w4:errorcluster)  [unwired: 9 in]
  n131 = disable-structure shown="RUN_TIME_ENGINE==True" {
    disable-tunnel: w4 -> [_ _]
    frame condition #0 (active) {
    }
    frame condition #1 {
      # "Call Quit LabVIEW if running as a built application."
      n132 = Quit LabVIEW() -> ()  [unwired: 1 in]
    }
  }
